vi "Get Vantage Lon V.vi"(8 "error in (no error)":errorcluster, 11 "longitude":T1) -> (0 "error out":errorcluster, 2 "function return":i16, 3 "longitude out":T1)   [LabVIEW 2009, in "VantagePro.lvlib"]
doc: "DllAccess short int _stdcall GetVantageLon_V ( LatLonValue *longitude);"
uses:
  VantagePro.lvlib
  <userlib>/VantagePro/VantagePro.dll
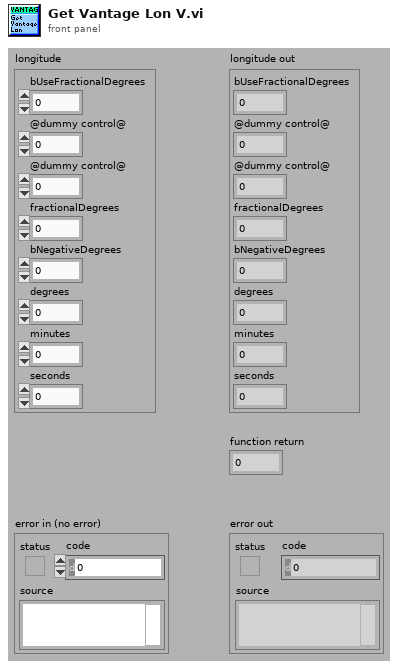
[diagram p1: front panel]
types:
  T1 = cluster{"bUseFractionalDegrees":i16, "@dummy control@":i8, "@dummy control@":i8, "fractionalDegrees":sgl, "bNegativeDegrees":i16, "degrees":i16, "minutes":i16, "seconds":i16}
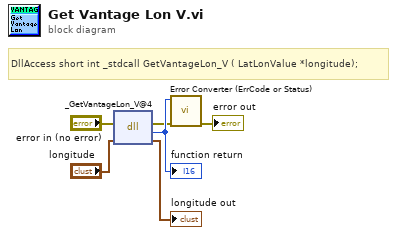
[diagram p0: block diagram]
diagram:
  # "DllAccess short int _stdcall GetVantageLon_V ( LatLonValue *longitude);"
  n1 = dll-call lib="C:/Program Files/National Instruments/LabVIEW 2010/user.lib/VantagePro/VantagePro.*" fn="_GetVantageLon_V@4"(error in="error in (no error)", "longitude"="longitude") -> (error out=w2:errorcluster, w6:i16, "longitude"=→"longitude out":T1)  [unwired: 2 in, 1 out]
  "function return" <- w6
  n2 = call "Error Converter (ErrCode or Status).vi"("error in (no error)"=w2, "error code"=w6) -> ("error out"=→"error out":errorcluster)  [unwired: 9 in]
